vi "UpImgCtrl.vi"(7 "Action":enum16{"Initial", "read", "release"}(ring)=enum."release", 8 "error in (no error)":errorcluster, 10 "GrayImg 2":T1, 11 "ColorImg 2":T2=enum."CUpSource") -> (0 "error out":errorcluster, 2 "GrayImg":string, 3 "ColorImg":string)   [LabVIEW 2019]
uses:
  Ctrl/UpColorImg.ctl
  Ctrl/UpGrayImg.ctl
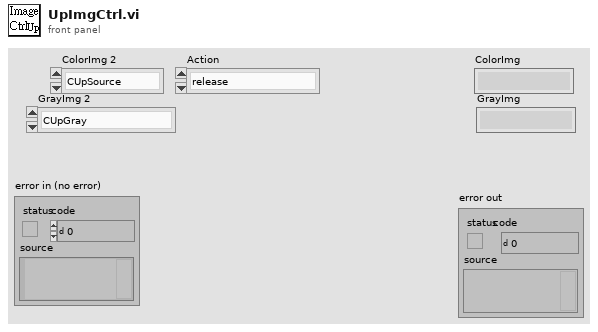
[diagram p1: front panel]
types:
  T1 = typedef "UpGrayImg.ctl" = enum16{"CUpGray", "CUpProce1", "CUpProce2", "UpPattern1", "UpPattern2", "UpCalibImg", "UpPreProcess"}
  T2 = typedef "UpColorImg.ctl" = enum16{"CUpCam", "CUpSource", "CUpShow", "CUpToProcess1", "CUpToProcess2", "CUpForMatch", "CUpForCheckNumbers", "CupPreProcess"}
  T3 = typedef "Image Type" = u32
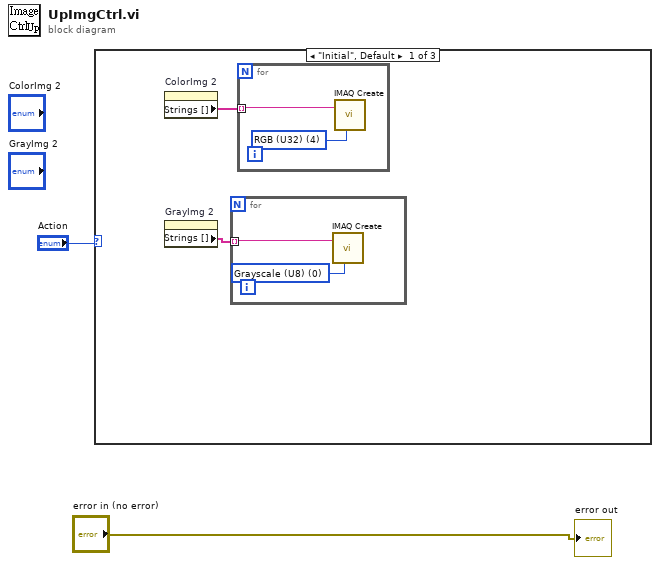
[diagram p0: block diagram]
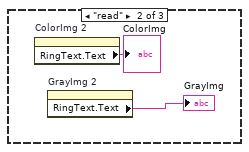
[diagram p2: hidden frame]
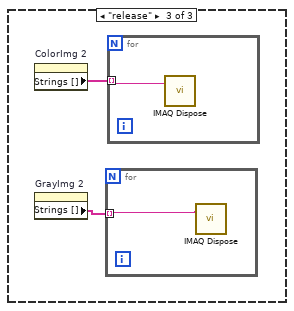
[diagram p3: hidden frame]
diagram:
  n1 = case shown="\"Initial\", Default" "Action" {
    frame "Initial", Default {
      n2 = property on="ColorImg 2" class="Enum (strict)"() -> ("Strings []"=w4:string[])  [unwired: 2 in, 2 out]
      n3 = property on="GrayImg 2" class="Enum (strict)"() -> ("Strings []"=w3:string[])  [unwired: 2 in, 2 out]
      n4 = for {
        tunnel: w3 -> [w6] mode=indexing
        w5 = T3 0 items=["Grayscale (U8)", "Grayscale (I16)", "Grayscale (SGL)", "Complex (CSG)", "RGB (U32)", "HSL (U32)", "RGB (U64)", "Grayscale (U16)"] ("Image Type")
        n5 = call "IMAQ Create"("Image Name"=w6, "Image Type"=w5) -> ()  [unwired: 3 in, 2 out]
      }
      n6 = for {
        tunnel: w4 -> [w8] mode=indexing
        w7 = T3 4 items=["Grayscale (U8)", "Grayscale (I16)", "Grayscale (SGL)", "Complex (CSG)", "RGB (U32)", "HSL (U32)", "RGB (U64)", "Grayscale (U16)"] ("Image Type")
        n7 = call "IMAQ Create"("Image Name"=w8, "Image Type"=w7) -> ()  [unwired: 3 in, 2 out]
      }
    }
    frame "read" {
      n8 = property on="ColorImg 2" class="Enum (strict)"() -> ("RingText.Text"=→"ColorImg":string)  [unwired: 2 in, 2 out]
      n9 = property on="GrayImg 2" class="Enum (strict)"() -> ("RingText.Text"=→"GrayImg":string)  [unwired: 2 in, 2 out]
    }
    frame "release" {
      n10 = property on="ColorImg 2" class="Enum (strict)"() -> ("Strings []"=w12:string[])  [unwired: 2 in, 2 out]
      n11 = property on="GrayImg 2" class="Enum (strict)"() -> ("Strings []"=w11:string[])  [unwired: 2 in, 2 out]
      n12 = for {
        tunnel: w11 -> [w13] mode=indexing
        n13 = call "IMAQ Dispose"("Image"=w13) -> ()  [unwired: 5 in, 1 out]
      }
      n14 = for {
        tunnel: w12 -> [w14] mode=indexing
        n15 = call "IMAQ Dispose"("Image"=w14) -> ()  [unwired: 5 in, 1 out]
      }
    }
  }
  "error out" <- "error in (no error)"
